vi "Destroy.vi"(8 "Error In":errorcluster, 11 "reference in":refnum<class "SDO Manager.lvclass">) -> (0 "Error Out":errorcluster, 3 "reference out":refnum<class "SDO Manager.lvclass">)   [LabVIEW 2024, in "CANopen Master.lvlib" / "SDO Manager.lvclass"]
uses:
  SDO Manager.lvclass
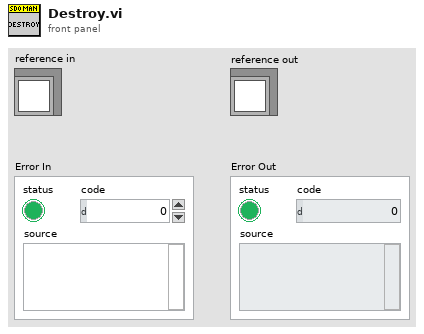
[diagram p1: front panel]
types:
  T1 = typedef "CANopen Master.lvlib/SDO Manager.lvclass/ObjectAttributes.ctl" = cluster{"SDO Response Map":map{u32, refnum<notifier>}}
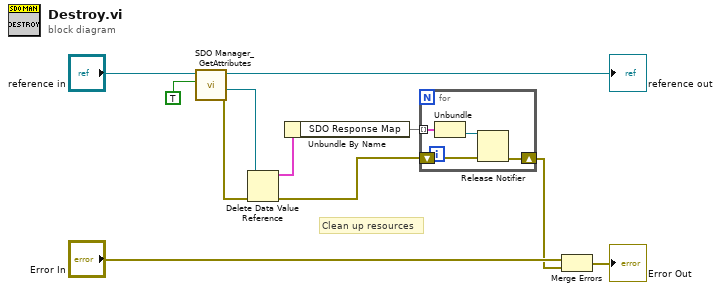
[diagram p0: block diagram]
diagram:
  # "Clean up resources"
  n1 = call "SDO Manager_GetAttributes.vi"("OnlyGetDvrReference(False)"=TRUE, "reference in"="reference in") -> ("Error Out"=w8:errorcluster, "DataRef"=w7:refnum<data-value>, "reference out"=→"reference out":refnum<class "SDO Manager.lvclass">)  [unwired: 6 in, 1 out]
  n2 = Delete Data Value Reference(data value reference=w7, error in=w8) -> (data value=w4:T1, error out=w2:errorcluster)
  n3 = Unbundle By Name(w4) -> ("SDO Response Map"=w3:map{u32, refnum<notifier>})
  n4 = for {
    tunnel: w3 -> [w15] mode=indexing
    shift-right: [w12] -> w1
    shift-left: w2 -> [w13]
    n5 = Unbundle(w15) -> ("Notifier"=w14:refnum<notifier>)  [unwired: 1 out]
    n6 = Release Notifier(notifier=w14, error in (no error)=w13) -> (error out=w12:errorcluster)  [unwired: 1 in, 2 out]
  }
  n7 = Merge Errors("Error In", w1) -> (→"Error Out":errorcluster)
